vi "Execute.vi"(8 "error in (no error)":errorcluster, 11 "Generic Driver in":refnum<class "Generic Driver.lvclass">) -> (0 "error out":errorcluster, 3 "Generic Driver out":refnum<class "Generic Driver.lvclass">)   [LabVIEW 2020, in "OOP.lvlib" / "Generic Driver.lvclass"]
uses:
  Generic Driver.lvclass
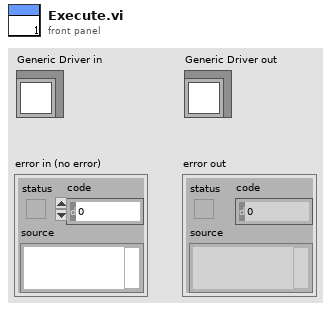
[diagram p1: front panel]
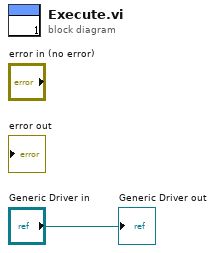
[diagram p0: block diagram]
diagram:
  "Generic Driver out" <- "Generic Driver in"
